vi "Export image.vi"(6 "Target":enum32{"File", "Clipboard"}(ring), 7 "File Type":enum32{"BMP", "EPS", "EMF", "PICT"}(ring), 9 "Graph reference":refnum<vi>, 10 "Folder selection":path, 11 "VI caller":refnum<vi>) -> (3 "Ready?":bool)   [LabVIEW 2021]
panel:
  in  "Hide Grid":bool
  in  "Export":bool
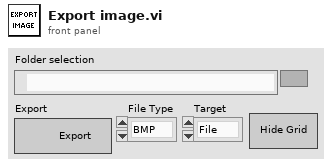
[diagram p1: front panel]
types:
  T1 = enum32{"Invalid", "Standard", "Closed", "Hidden", "Minimized", "Maximized"}
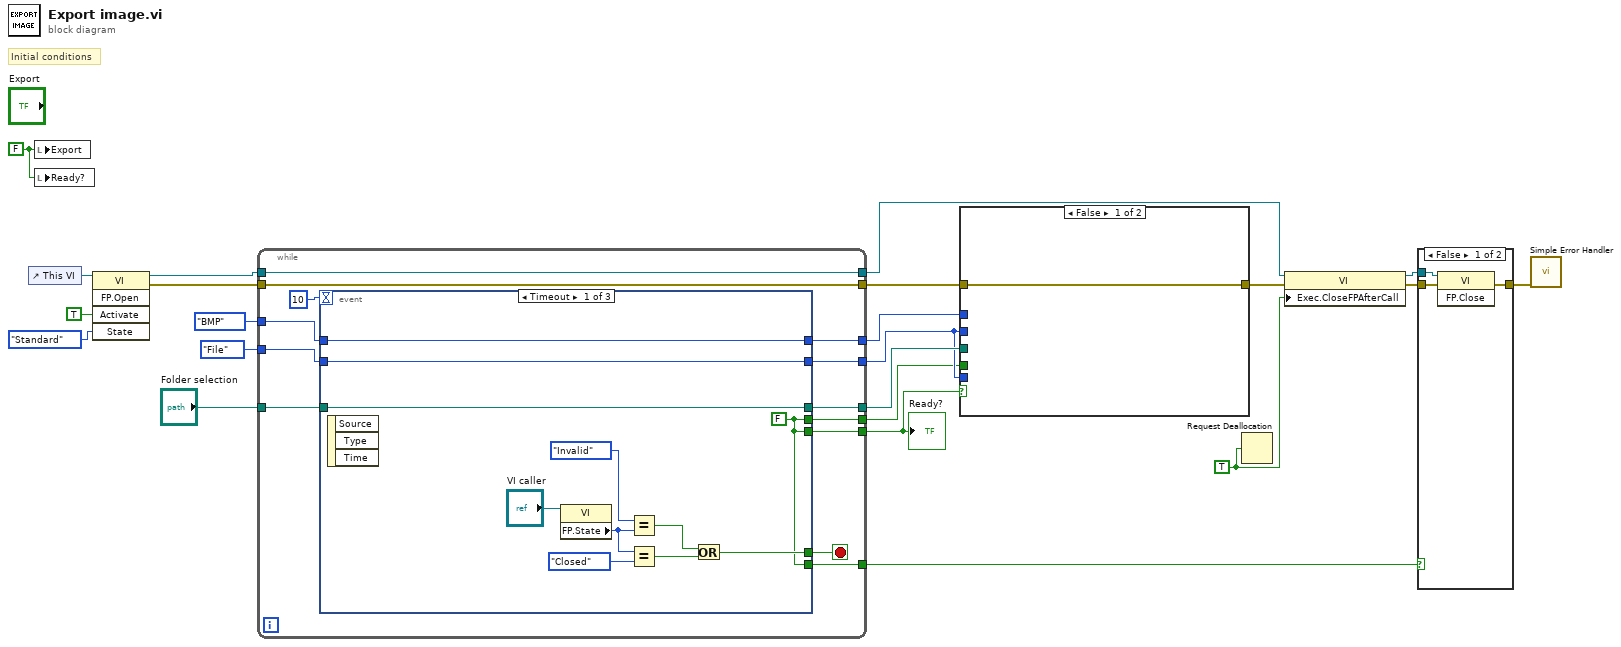
[diagram p0: block diagram]
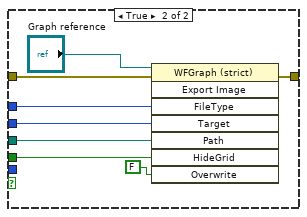
[diagram p3: hidden frame]
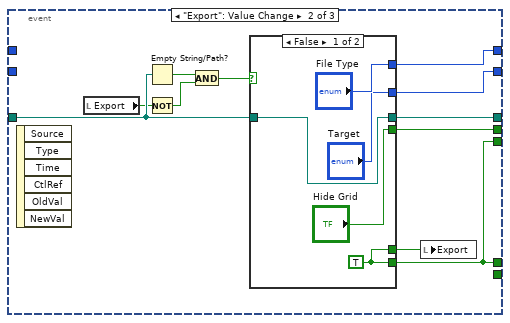
[diagram p4: hidden frame]
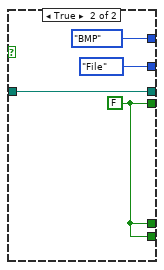
[diagram p5: hidden frame]
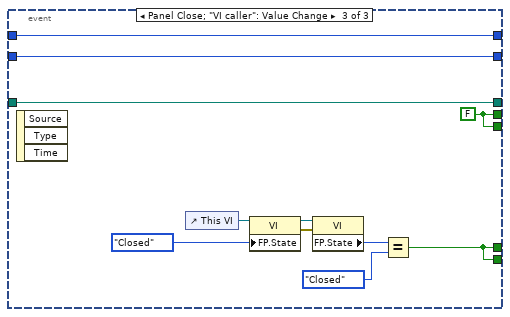
[diagram p6: hidden frame]
diagram:
  w6 = TRUE ("Activate?")
  w14 = FALSE
  # "Initial conditions"
  n1 = control-ref of="This VI"() -> (w3:refnum<vi>)
  n2 = local write "Export"(w14) -> ()
  n3 = local write "Ready?"(w14) -> ()
  n4 = invoke on="Invoke Node" class="VI" method="FP.Open"(reference=w3, "Activate"=TRUE ("Activate?"), "State"=T1."Standard") -> (reference out=w20:refnum<vi>, error out=w21:errorcluster)  [unwired: 2 in, 3 out]
  n5 = while {
    tunnel: [w27] -> w11
    tunnel: w21 -> [w35]
    tunnel: w20 -> [w34]
    tunnel: [w34] -> w18
    tunnel: [w35] -> w17
    tunnel: "Folder selection" -> [w32]
    tunnel: [w31] -> w10
    tunnel: [w30] -> w8
    tunnel: [w29] -> w9
    tunnel: [w28] -> w7
    tunnel: [w25] -> w12
    tunnel: enum32{"BMP", "EPS", "EMF", "PICT"}."BMP" ("File Type") -> [w24]
    tunnel: enum32{"File", "Clipboard"}."File" ("Target") -> [w23]
    stop <- w33 stop-if-true
    n6 = event shown="[0] Timeout" {
      selector: _ -> [_ _ _]
      dyn-events: _ -> [_ _ _]
      timeout: 10 -> [_ _ _]
      tunnel: [w42 w47 w74] -> w33
      tunnel: w32 -> [w38 w57 w75]
      tunnel: [w38 w56 w75] -> w31
      tunnel: [w40 w55 w68] -> w30
      tunnel: [w39 w54 w67] -> w29
      tunnel: [w41 w53 w69] -> w28
      tunnel: [w41 w47 w69] -> w27
      tunnel: [w41 _ w74] -> w25
      tunnel: w24 -> [w40 _ w68]
      tunnel: w23 -> [w39 _ w67]
      event Timeout {
        w41 = FALSE
        n7 = event-data() -> ()  [unwired: 1 in, 3 out]
        n8 = property class="VI"(reference="VI caller") -> ("FP.State"=w36:T1)  [unwired: 1 in, 2 out]
        n9 = Equal?(x=T1."Invalid" ("Front Panel Window:State"), y=w36) -> (x = y?=w44:bool)
        n10 = Equal?(x=w36, y=T1."Closed" ("Front Panel Window:State")) -> (x = y?=w43:bool)
        n11 = Or(x=w44, y=w43) -> (x .or. y?=w42:bool)
      }
      event "Export": Value Change {
        n12 = event-data() -> ()  [unwired: 1 in, 6 out]
        n13 = local read "Export"() -> (w50:bool)
        n14 = Empty String/Path?(string/path=w57) -> (empty?=w52:bool)
        n15 = Not(x=w50) -> (.not. x?=w49:bool)
        n16 = And(x=w52, y=w49) -> (x .and. y?=w51:bool)
        n17 = case shown="False" w51 {
          tunnel: w57 -> [w62 w65]
          tunnel: [w62 w65] -> w56
          tunnel: ["File Type" enum32{"BMP", "EPS", "EMF", "PICT"}."BMP" ("File Type")] -> w55
          tunnel: ["Target" enum32{"File", "Clipboard"}."File" ("Target")] -> w54
          tunnel: ["Hide Grid" w63] -> w53
          tunnel: [w58 w63] -> w47
          tunnel: [w58 w63] -> w48
          frame False {
            w58 = TRUE
          }
          frame True {
            w63 = FALSE ("Hide Grid")
          }
        }
        n18 = local write "Export"(w48) -> ()
      }
      event Panel Close; "VI caller": Value Change {
        w69 = FALSE ("Hide Grid")
        n19 = event-data() -> ()  [unwired: 1 in, 3 out]
        n20 = control-ref of="This VI"() -> (w72:refnum<vi>)
        n21 = property class="VI"(reference=w72, "FP.State"=T1."Closed" ("Front Panel Window:State")) -> (reference out=w71:refnum<vi>, error out=w70:errorcluster)  [unwired: 1 in]
        n22 = property class="VI"(reference=w71, error in=w70) -> ("FP.State"=w77:T1)  [unwired: 2 out]
        n23 = Equal?(x=w77, y=T1."Closed" ("Front Panel Window:State")) -> (x = y?=w74:bool)
      }
    }
  }
  "Ready?" <- w11
  n24 = case shown="False" w11 {
    tunnel: w17 -> [w78 w86]
    tunnel: w9 -> [_ _]
    tunnel: w10 -> [_ w84]
    tunnel: w9 -> [_ w83]
    tunnel: w8 -> [_ w82]
    tunnel: w7 -> [_ w81]
    tunnel: [w78 w79] -> w5
    frame False {
    }
    frame True {
      n25 = invoke on="Invoke Node" class="WFGraph (strict)" method="Export Image"(reference="Graph reference", error in=w86, "FileType"=w82, "Target"=w83, "Path"=w84, "HideGrid"=w81, "Overwrite"=FALSE ("Always Overwrite")) -> (error out=w79:errorcluster)  [unwired: 1 in, 7 out]
    }
  }
  n26 = Request Deallocation(w6) -> ()
  n27 = property class="VI"(reference=w18, error in=w5, "Exec.CloseFPAfterCall"=w6) -> (reference out=w16:refnum<vi>, error out=w15:errorcluster)
  n28 = case shown="False" w12 {
    tunnel: [w89 w90] -> w4
    tunnel: w16 -> [w88 _]
    tunnel: w15 -> [w87 w90]
    frame False {
      n29 = invoke class="VI" method="FP.Close"(reference=w88, error in=w87) -> (error out=w89:errorcluster)  [unwired: 1 in, 2 out]
    }
    frame True {
    }
  }
  n30 = call <vilib>:"Simple Error Handler.vi"("error in (no error)"=w4) -> ()  [unwired: 4 in, 5 out]
